vi "GFITS_WriteHeaders.vi"(1 "Database RefNum in":T1, 5 "ref":u64, 7 "number of extensions":u16, 9 "Keywords":string[][][](array[string]), 11 "number of keywords":i32[](array[numeric]), 12 "expID in":string) -> (6 "ref out":u64, 10 "expID":string)   [LabVIEW 2016]
uses:
  DBSHAND/private/vis/DatabaseHand_RefNum.ctl
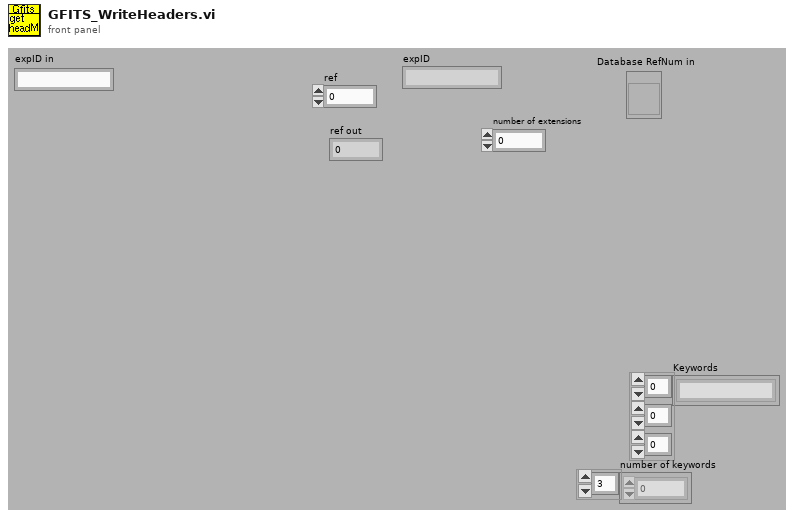
[diagram p1: front panel]
types:
  T1 = typedef "DatabaseHand_RefNum.ctl" = refnum<vi>
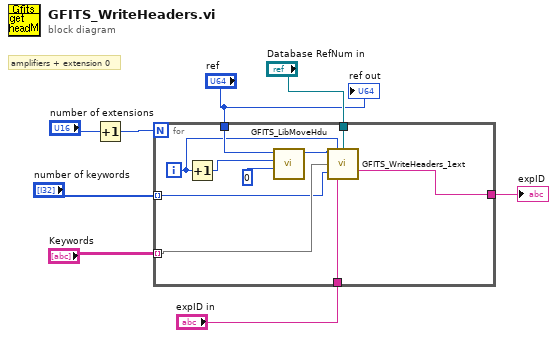
[diagram p0: block diagram]
diagram:
  # "amplifiers + extension 0"
  n1 = Increment(x="number of extensions") -> (x+1=w7:u16)
  n2 = for {
    N: w7 -> [_]
    tunnel: "number of keywords" -> [w14] mode=indexing
    tunnel: "ref" -> [w18]
    tunnel: "Keywords" -> [w15] mode=indexing
    tunnel: "Database RefNum in" -> [w11]
    tunnel: [w10] -> w3
    tunnel: "expID in" -> [w9]
    i -> [w12]
    n3 = Increment(x=w12) -> (x+1=w13:i32)
    n4 = call "GFITS_LibMoveHdu.vi"("hdutype"=0, "hdunum"=w13, "ref"=w18) -> ("ref out"=w16:u64)  [unwired: 1 in, 7 out]
    n5 = call "GFITS_WriteHeaders_1ext.vi"("ref"=w16, "extension"=w12, "Database RefNum in"=w11, "Keywords"=w15, "numer of keywords"=w14, "expID in"=w9) -> ("expID"=w10:string)  [unwired: 1 in, 8 out]
  }
  "expID" <- w3
  "ref out" <- "ref"
